vi "Report_A131258.vi"(6 "文件重命名":bool, 7 "文件名称":string, 8 "错误输入（无错误）":errorcluster, 11 "布尔数组":bool[][](array[boolean])=[[TRUE]]) -> (0 "error out":errorcluster caption="错误输出")   [LabVIEW 2020]
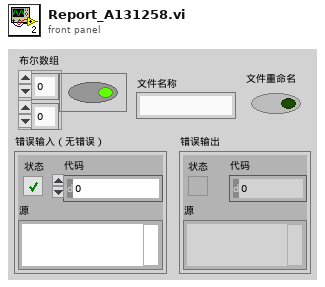
[diagram p1: front panel]
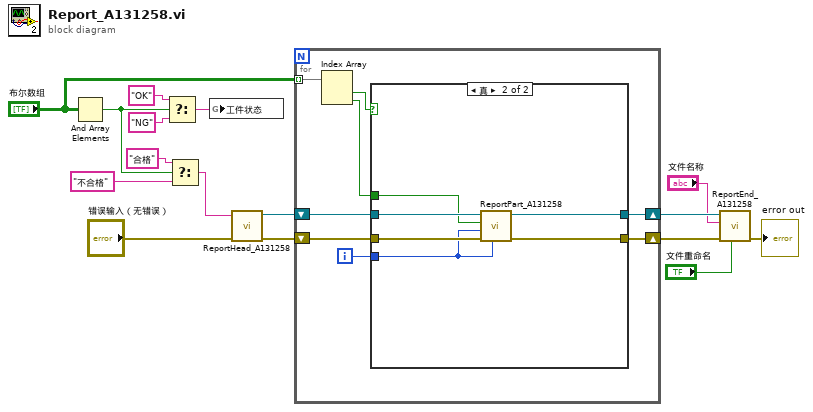
[diagram p0: block diagram]
diagram:
  n1 = And Array Elements(Boolean array="布尔数组") -> (logical AND=w2:bool)
  n2 = Select(t="OK", s=w2, f="NG") -> (s? t:f=w1:string)
  n3 = Select(t="合格", s=w2, f="不合格") -> (s? t:f=w5:string)
  n4 = global write "追溯全部变量.vi" "工件状态"(w1) -> ()
  n5 = call "ReportHead_A131258.vi"("error in (no error)"="错误输入（无错误）", "产品状态"=w5) -> ("error out"=w15:errorcluster, "report out"=w16:refnum<class "NI_report.lvclass">)  [unwired: 8 in]
  n6 = for {
    shift-right: [w22] -> w14
    shift-left: w16 -> [w24]
    shift-right: [w21] -> w13
    shift-left: w15 -> [w23]
    tunnel: "布尔数组" -> [w19] mode=indexing
    i -> [w20]
    n7 = Index Array(array=w19) -> (element #1=w18:bool, element #2=w17:bool)  [unwired: 2 in]
    n8 = case shown="真" w18 {
      tunnel: w24 -> [w25 w32]
      tunnel: w23 -> [w26 w31]
      tunnel: [w25 w30] -> w22
      tunnel: [w26 w29] -> w21
      tunnel: w20 -> [_ w27]
      tunnel: w17 -> [_ w28]
      frame False {
      }
      frame True {
        n9 = call "ReportPart_A131258.vi"("试验项目"=w27, "error in"=w31, "索引"=w27, "合格"=w28, "report in"=w32) -> ("error out 2"=w29:errorcluster, "report out"=w30:refnum<class "NI_report.lvclass">)  [unwired: 5 in]
      }
    }
  }
  n10 = call "ReportEnd_A131258.vi"("文件重命名"="文件重命名", "error in (no error)"=w13, "文件名称"="文件名称", "report in"=w14) -> ("error out"=→"error out":errorcluster)  [unwired: 7 in]
